vi "getI32[]Value.vi"(7 "Name":string, 8 "error in (no error)":errorcluster, 11 "tBSONDocument in":refnum<class "tBSONDocument.lvclass">) -> (0 "error out":errorcluster, 2 "Value":i32[](array[numeric]), 3 "tBSONDocument out":refnum<class "tBSONDocument.lvclass">)   [LabVIEW 2013, in "BSON.lvlib" / "tBSONDocument.lvclass"]
doc: "Retrieves an array of I32s from a BSON document."
uses:
  tBSONDocument.lvclass
  BSONElements/tBSONArray/tBSONArray.lvclass
  BSONElements/tBSON_I32/tBSON_I32.lvclass
  BSONElements/tBSONArray/getValue.vi
  BSONElements/tBSON_I32/getValue.vi
  tBSONElement/tBSONElement.lvclass
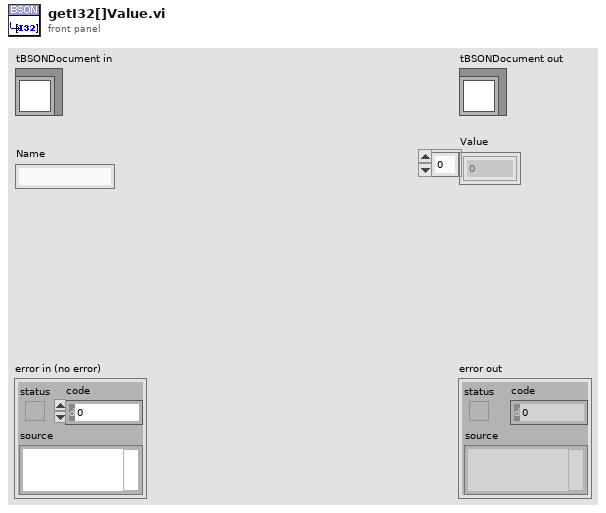
[diagram p1: front panel]
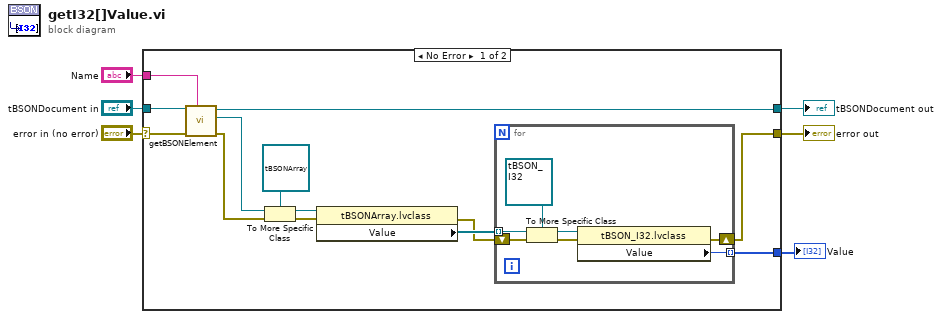
[diagram p0: block diagram]
diagram:
  n1 = case shown="No Error" "error in (no error)" {
    selector: "error in (no error)" -> [w19 w28]
    tunnel: [w10 w28] -> w2
    tunnel: [w18 w27] -> w3
    tunnel: [w9 _] -> w1
    tunnel: "tBSONDocument in" -> [w8 w27]
    tunnel: "Name" -> [w7 _]
    frame No Error {
      n2 = call "getBSONElement.vi"("Name"=w7, "error in (no error)"=w19, "tBSONDocument in"=w8) -> ("error out"=w15:errorcluster, "Element"=w16:refnum<class "tBSONElement.lvclass">, "tBSONDocument out"=w18:refnum<class "tBSONDocument.lvclass">)  [unwired: 6 in]
      n3 = To More Specific Class(target class=refnum<class "tBSONArray.lvclass"> refnum ("BSON.lvlib:tBSONArray.lvclass"), reference=w16, error in=w15) -> (specific class reference=w14:refnum<class "tBSONArray.lvclass">, error out=w13:errorcluster)
      n4 = property class="tBSONArray.lvclass"(reference=w14, error in=w13) -> (error out=w11:errorcluster, "Value"=w12:refnum<class "tBSONElement.lvclass">[])  [unwired: 1 out]
      n5 = for {
        tunnel: w12 -> [w25] mode=indexing
        shift-right: [w22] -> w10
        shift-left: w11 -> [w26]
        tunnel: [w21] -> w9 mode=indexing
        n6 = To More Specific Class(target class=refnum<class "tBSON_I32.lvclass"> refnum ("lvMongoDriver.lvlib:BSON.lvlib:tBSON_I32.lvclass"), reference=w25, error in=w26) -> (specific class reference=w24:refnum<class "tBSON_I32.lvclass">, error out=w23:errorcluster)
        n7 = property class="tBSON_I32.lvclass"(reference=w24, error in=w23) -> (error out=w22:errorcluster, "Value"=w21:i32)  [unwired: 1 out]
      }
    }
    frame Error {
    }
  }
  "error out" <- w2
  "tBSONDocument out" <- w3
  "Value" <- w1
